vi "ExportBadDependencies.vi"(8 "error in (no error)":errorcluster, 10 "IExporter":refnum<class "IExporter.lvclass">, 11 "CReporter in":refnum<class "CReporter.lvclass">) -> (0 "error out":errorcluster, 3 "CReporter out":refnum<class "CReporter.lvclass">)   [LabVIEW 2020, in "DependencyInspection.lvlib" / "CReporter.lvclass"]
uses:
  CReporter.lvclass
  CDependencyList/CDependencyList.lvclass
  obj/Addons/ExtensionInterfaces.lvlibp/IExporter/ExportType.ctl
  obj/Addons/ExtensionInterfaces.lvlibp/IExporter/IExporter.lvclass
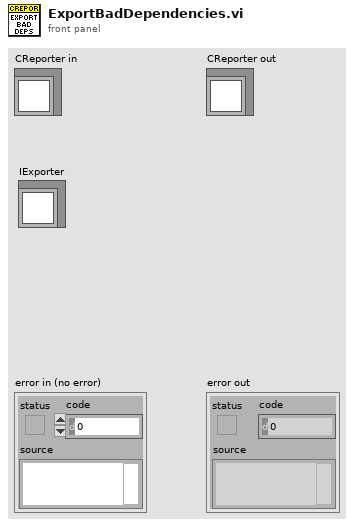
[diagram p1: front panel]
types:
  T1 = typedef "ExtensionInterfaces.lvlibp/IExporter.lvclass/ExportType.ctl" = enum16{"Dependencies", "Rules", "Invalid dependencies", "Concessions", "Undeclared"}
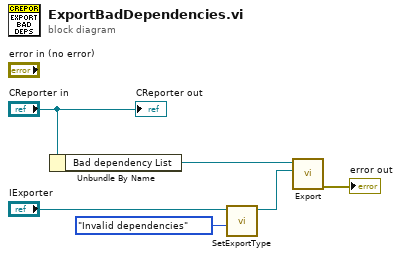
[diagram p0: block diagram]
diagram:
  n1 = Unbundle By Name("CReporter in") -> ("Bad dependency List"=w5:refnum<class "CDependencyList.lvclass">)
  n2 = call-dynamic "SetExportType.vi"("Export type"=ExportType."Invalid dependencies", "IExporter in"="IExporter") -> ("IExporter out"=w1:refnum<class "IExporter.lvclass">)  [unwired: 8 in, 1 out]
  n3 = call-dynamic "Export.vi"("IExporter"=w1, "CDependencyList in"=w5) -> ("error out"=→"error out":errorcluster)  [unwired: 8 in, 1 out]
  "CReporter out" <- "CReporter in"
